vi "Get Control State.vi"(7 "ATM State":T1, 10 "Controls":T2) -> (2 "Enable State":T3(ring))   [LabVIEW 2020, in "ATM View Model.lvclass"]
uses:
  ATM View Model.lvclass
  Controls.ctl
  ATM Controller/State.ctl
  ATM Controller/ATM Controller.lvclass
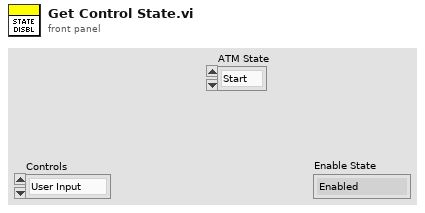
[diagram p1: front panel]
types:
  T1 = typedef "ATM Controller.lvclass/State.ctl" = enum16{"Start", "Insert Card", "Deposit", "Withdraw", "Fast Cash", "None", "Balance Inquiry", "Return Card"}
  T2 = typedef "ATM View Model.lvclass/Controls.ctl" = enum16{"User Input", "Enter", "Left Menu", "Righ Menu", "Left Button", "Right Button", "Card Simulator"}
  T3 = enum8{"Enabled", "Disabled", "Disabled and Grayed Out"}
  T4 = map{cluster{"ATM State":T1, "Controls":T2}, enum8{"Enabled", "Disabled", "Disabled and Grayed Out"}}
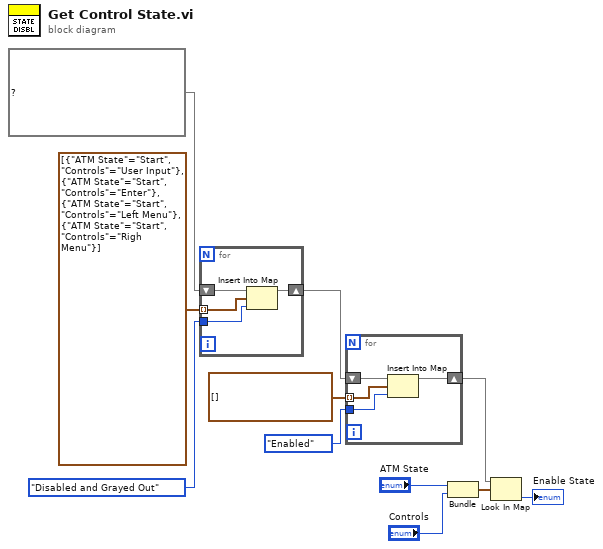
[diagram p0: block diagram]
diagram:
  n1 = for {
    tunnel: cluster{"ATM State":T1, "Controls":T2}[] [{"ATM State"=enum."Start", "Controls"=enum."User Input"}, {"ATM State"=enum."Start", "Controls"=enum."Enter"}, {"ATM State"=enum."Start", "Controls"=enum."Left Menu"}, {"ATM State"=enum."Start", "Controls"=enum."Righ Menu"}] ("key") -> [w13] mode=indexing
    shift-right: [w14] -> w4
    shift-left: T4 {} ("map") -> [w15]
    tunnel: T3."Disabled and Grayed Out" ("Enable State") -> [w12]
    n2 = Insert Into Map(map in=w15, key=w13, value=w12) -> (map out=w14:T4)  [unwired: 2 out]
  }
  n3 = for {
    tunnel: cluster{"ATM State":T1, "Controls":T2}[] [] ("key") -> [w17] mode=indexing
    shift-right: [w18] -> w3
    shift-left: w4 -> [w19]
    tunnel: T3."Enabled" ("Enable State") -> [w16]
    n4 = Insert Into Map(map in=w19, key=w17, value=w16) -> (map out=w18:T4)  [unwired: 2 out]
  }
  n5 = Bundle("ATM State"="ATM State", "Controls"="Controls") -> (w8:cluster{"ATM State":T1, "Controls":T2})  [unwired: 1 in]
  n6 = Look In Map(map=w3, key=w8) -> (value=→"Enable State":T3)  [unwired: 1 in, 1 out]
